vi "SIFS_ReadPosition.vi"(2 "FATOR":dbl, 3 "ID":string, 4 "VISA resource name":refnum<visa-resource-name>) -> (0 "error out":errorcluster, 1 "Position":dbl)   [LabVIEW 2018]
panel:
  out "output 3":string
  out "output 2":string
  out "output 1":string
  out "NumPosicao":i32
  out "StrPosicao":string
  out "StrComando":string
  out "read buffer":string
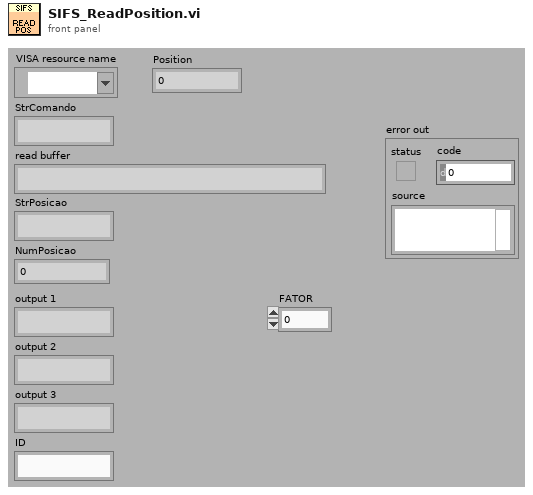
[diagram p1: front panel]
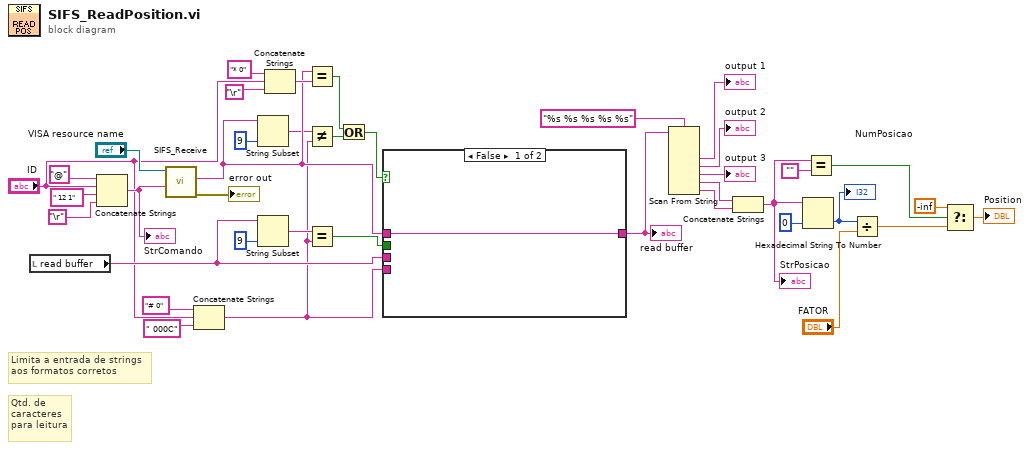
[diagram p0: block diagram]
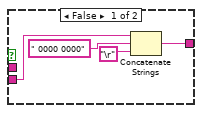
[diagram p3: hidden frame]
diagram:
  # "Limita a entrada de strings\naos formatos corretos"
  # "Qtd. de\ncaracteres\npara leitura"
  n1 = local read "read buffer"() -> (w27:string)
  n2 = Concatenate Strings("@" ("string"), "ID", " 12 1", "\r") -> (w38:string)
  "StrComando" <- w38
  n3 = call "SIFS_Receive.vi"("Command to SIFS"=w38, "VISA resource name"="VISA resource name") -> ("error out"=→"error out":errorcluster, "Response from SIFS"=w23:string)  [unwired: 2 in, 2 out]
  n4 = Concatenate Strings("# 0" ("string"), "ID", " 000C") -> (w3:string)
  n5 = String Subset(string=w23, length (rest)=9 ("length (rest)")) -> (substring=w22:string)  [unwired: 1 out]
  n6 = String Subset(string=w27, length (rest)=9 ("length (rest)")) -> (substring=w29:string)  [unwired: 1 out]
  n7 = Concatenate Strings("* 0" ("string"), "ID", "\r") -> (w25:string)
  n8 = Equal?(x=w23, y=w25) -> (x = y?=w21:bool)
  n9 = Not Equal?(x=w22, y=w3) -> (x != y?=w20:bool)
  n10 = Equal?(x=w29, y=w3) -> (x = y?=w28:bool)
  n11 = Or(x=w21, y=w20) -> (x .or. y?=w19:bool)
  n12 = case shown="False" w19 {
    tunnel: [w40 w44] -> w1
    tunnel: w28 -> [_ w42]
    tunnel: w27 -> [_ w43]
    tunnel: w23 -> [w40 _]
    tunnel: w3 -> [_ w41]
    frame False {
    }
    frame True {
      n13 = case shown="True" w42 {
        tunnel: [w48 w49] -> w44
        tunnel: w43 -> [_ w49]
        tunnel: w41 -> [w45 _]
        frame False {
          n14 = Concatenate Strings(w45, " 0000 0000", "\r") -> (w48:string)
        }
        frame True {
        }
      }
    }
  }
  "read buffer" <- w1
  n15 = Scan From String(format string="%s %s %s %s %s", input string=w1) -> (output 1=→"output 1":string, output 2=→"output 2":string, output 3=→"output 3":string, output 4=w35:string, output 5=w34:string)  [unwired: 2 in, 8 out]
  n16 = Concatenate Strings(w35, w34) -> (w6:string)
  "StrPosicao" <- w6
  n17 = Hexadecimal String To Number(string=w6, default (0uL)=0 ("default (0 U32)")) -> (number=w11:i32)  [unwired: 2 out]
  "NumPosicao" <- w11
  n18 = Equal?(x=w6, y="") -> (x = y?=w9:bool)
  n19 = Divide(x=w11, y="FATOR") -> (x/y=w5:dbl)
  n20 = Select(t=-inf, s=w9, f=w5) -> (s? t:f=→"Position":dbl)
